vi "SPD.HV_Bias SubTest.vi"(0 "SPD.Stand Ctrl in":T3 {"spdDeviceSession"."hidSPD.Controller"."HV_bias" format="%#_6p, V"; "spdDeviceSession"."hidSPD.Controller"."TSet" format="%#_6p, DegC"}, 1 "Comparison Mode":T2, 5 "HV_values":dbl[](array[numeric]), 7 "Gate":dbl, 9 "range":T1, 11 "Error In":errorcluster, 12 "Progress":refnum<vi>, 13 "Graph":refnum<vi>) -> (4 "SPD.Stand Ctrl out":T3 {"spdDeviceSession"."hidSPD.Controller"."HV_bias" format="%#_6p, V"; "spdDeviceSession"."hidSPD.Controller"."TSet" format="%#_6p, DegC"}, 6 "last HV_bias":dbl, 8 "Clicks Count":dbl, 10 "result":bool, 15 "Error Out":errorcluster)   [LabVIEW 2018]
uses:
  typedefs/SPD.Stand Ctrl.ctl
  Instruments/SPD HID Interface/hidSPDLibForLabView/LibVIs/hidSPD Controls/hidSPD Device Session.ctl
  Instruments/SPD HID Interface/hidSPDLibForLabView/LibVIs/hidSPD Controls/hidSPD Controller.ctl
  Instruments/KC705 DevBoard/typedefs/DevB.Session.ctl
  Instruments/KeySight 53230A/typedefs/FreqC.Session.ctl
  Instruments/KeySight 8164B/KeySight 8164B LAN InstrLib/typedefs/KeySight 8164B control.ctl
  Instruments/LeCroy SDA830/typedefs/LeCroy.Session.ctl
  typedefs/SPD.Events.ctl
  <vilib>/Utility/config.llb/Config Data RefNum.ctl
  SubVIs/comparison mode.ctl
  SubVIs/Min_Max.ctl
  Instruments/SPD HID Interface/hidSPDLibForLabView/LibVIs/hidSPD Controls/hidSPD Controller Setup Report.ctl
  Instruments/SPD HID Interface/hidSPDLibForLabView/LibVIs/hidSPD Write Report/hidSPD Setup Controller.vi
  Instruments/SPD HID Interface/hidSPDLibForLabView/hidSPDLibForLabView.lvlib
  Instruments/KeySight 8164B/KeySight 8164B LAN InstrLib.lvlib
  <vilib>/Utility/config.llb/NI_LVConfig.lvlib
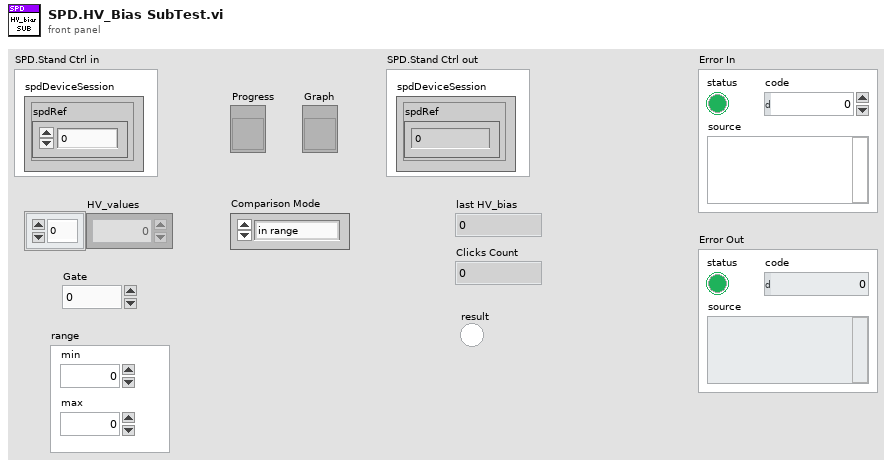
[diagram p1: front panel]
types:
  T1 = typedef "Min_Max.ctl" = cluster{"min":dbl, "max":dbl}
  T2 = typedef "comparison mode.ctl" = enum16{"in range", "bigger then min", "bigger then max", "less then min", "less then max"}
  T3 = typedef "SPD.Stand Ctrl.ctl" = cluster{"spdDeviceSession":T4, "DevBSession":T6, "FreqCSession":T7, "8164BSession":T8, "LeCroySession":T9, "Events":T10, "configFile":T11}
  T4 = typedef "hidSPDLibForLabView.lvlib/hidSPD Device Session.ctl" = cluster{"spdRef":u64, "connected":bool, "spdName":string, "hidSPD.Controller":T5}
  T5 = typedef "hidSPDLibForLabView.lvlib/hidSPD Controller.ctl" = cluster{"TSet":sgl, "HV_bias":sgl, "DDS_stb_code":u16}
  T6 = typedef "DevB.Session.ctl" = cluster{"DevBRef":refnum<visa-resource-name>, "connected":bool}
  T7 = typedef "FreqC.Session.ctl" = cluster{"FreqCRef":refnum<visa-resource-name>, "timeout":dbl, "connected":bool}
  T8 = typedef "KeySight 8164B LAN InstrLib.lvlib/KeySight 8164B control.ctl" = cluster{"Connection ID":refnum<k5>, "Connected":bool, "Info":string, "Slots Info":string[]}
  T9 = typedef "LeCroy.Session.ctl" = cluster{"LeCroySession":refnum<visa-resource-name>, "connected":bool}
  T10 = typedef "SPD.Events.ctl" = cluster{"DCRTest":refnum<user-event>, "Stop":refnum<user-event>}
  T11 = typedef "NI_LVConfig.lvlib/Config Data RefNum.ctl" = refnum<k1>
  T12 = typedef "hidSPDLibForLabView.lvlib/hidSPD Controller Setup Report.ctl" = cluster{"TSet":sgl, "HV_bias":sgl, "DDS_stb_code":u16, "SPD_reset":u16, "MCU_reset":u16}
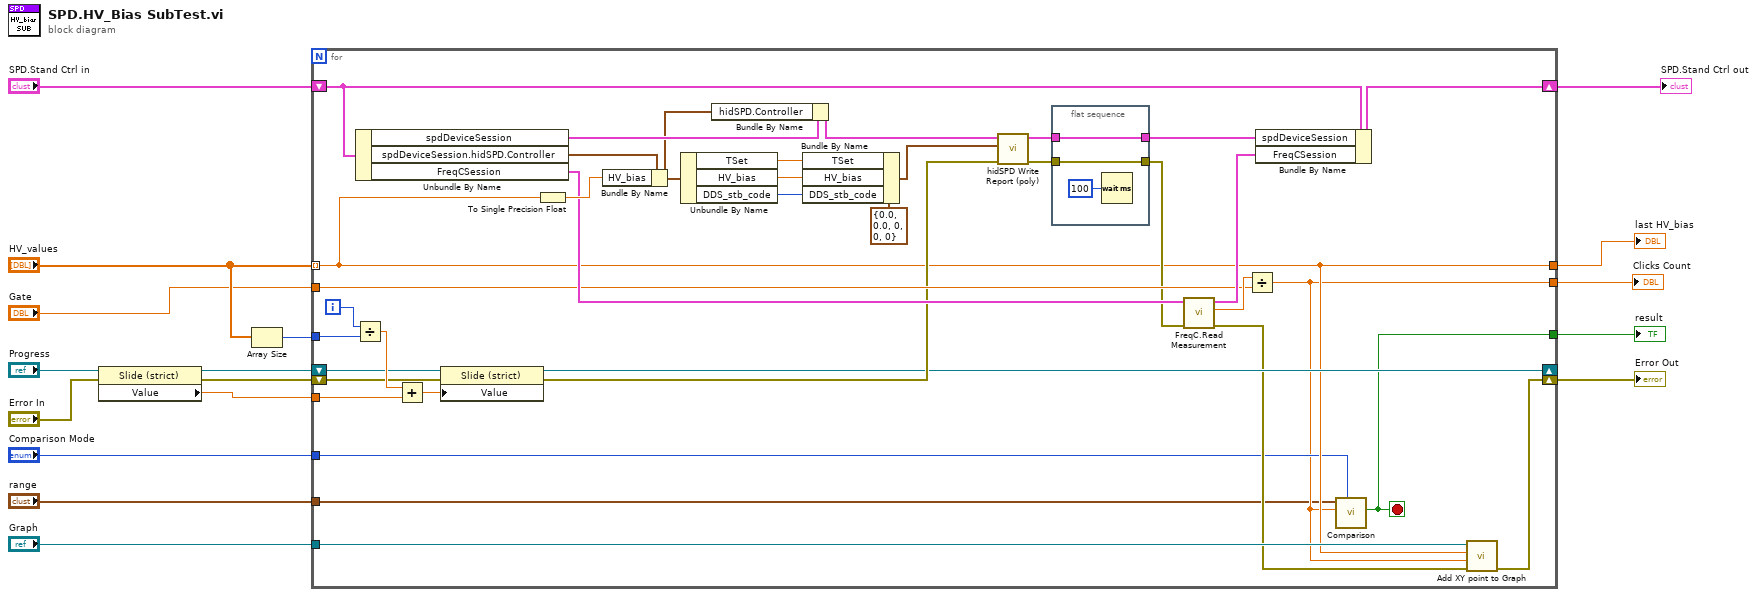
[diagram p0: block diagram]
diagram:
  n1 = property class="Slide (strict)"(reference="Progress", error in="Error In") -> (reference out=w8:refnum<vi>, error out=w6:errorcluster, "Value"=w5:dbl)
  n2 = Array Size(array="HV_values") -> (size(s)=w13:i32)
  n3 = for {
    shift-right: [w25] -> w15
    shift-left: w6 -> [w32]
    shift-right: [w43] -> w16
    shift-left: "SPD.Stand Ctrl in" -> [w47]
    tunnel: "HV_values" -> [w27] mode=indexing
    tunnel: "Gate" -> [w39]
    tunnel: [w24] -> w4
    tunnel: [w27] -> w2
    tunnel: w13 -> [w34]
    shift-right: [w30] -> _
    shift-left: w8 -> [w29]
    tunnel: "Graph" -> [w28]
    tunnel: [w22] -> w3
    tunnel: "Comparison Mode" -> [w23]
    tunnel: w5 -> [w20]
    tunnel: "range" -> [w18]
    i -> [w19]
    stop <- w24 stop-if-true
    n4 = Divide(x=w19, y=w34) -> (x/y=w33:dbl)
    n5 = Unbundle By Name(w47) -> ("spdDeviceSession"=w54:T4, "spdDeviceSession.hidSPD.Controller"=w52:T5, "FreqCSession"=w41:T7)
    n6 = Add(x=w33, y=w20) -> (x+y=w21:dbl)
    n7 = property class="Slide (strict)"(reference=w29, error in=w32, "Value"=w21) -> (reference out=w30:refnum<vi>, error out=w31:errorcluster)
    n8 = To Single Precision Float(number=w27) -> (single precision float=w42:sgl)
    n9 = Bundle By Name(cluster=w52, "HV_bias"=w42) -> (w45:T5)
    n10 = Unbundle By Name(w45) -> ("TSet"=w51:sgl, "HV_bias"=w50:sgl, "DDS_stb_code"=w49:u16)
    n11 = Bundle By Name(cluster=w54, "hidSPD.Controller"=w45) -> (w46:T4)
    n12 = Bundle By Name(cluster=T12 {"TSet"=0.0, "HV_bias"=0.0, "DDS_stb_code"=0, "SPD_reset"=0, "MCU_reset"=0} ("hidSPD Controller Setup report"), "TSet"=w51, "HV_bias"=w50, "DDS_stb_code"=w49) -> (w48:T12)
    n13 = call-poly "hidSPD Write Report (poly).vi"("error in (no error)"=w31, "hidSPD Controller Setup report"=w48, "spdDevSession in"=w46) -> ("error out"=w37:errorcluster, "spdDevSession out"=w38:T4)  [unwired: 7 in]
    n14 = flat-sequence {
      tunnel: [w57] -> w35
      tunnel: w38 -> [w57]
      tunnel: [w56] -> w36
      tunnel: w37 -> [w56]
      frame #0 {
        n15 = Wait (ms)(milliseconds to wait=u32 100) -> ()  [unwired: 1 out]
      }
    }
    n16 = call "FreqC.Read Measurement.vi"("error In"=w36, "FreqC Session in"=w41) -> ("error out"=w26:errorcluster, "Measurement"=w40:dbl, "FreqC Session out"=w44:T7)  [unwired: 7 in]
    n17 = Divide(x=w40, y=w39) -> (x/y=w22:dbl)
    n18 = Bundle By Name(cluster=w47, "spdDeviceSession"=w35, "FreqCSession"=w44) -> (w43:T3)
    n19 = call "Comparison.vi"("Comparison Mode"=w23, "value"=w22, "minMax"=w18) -> ("result"=w24:bool)  [unwired: 8 in]
    n20 = call "Add XY point to Graph.vi"("error in (no error)"=w26, "Y"=w22, "X"=w27, "Graph in"=w28) -> ("error out"=w25:errorcluster)  [unwired: 6 in, 1 out]
  }
  "SPD.Stand Ctrl out" <- w16
  "Error Out" <- w15
  "result" <- w4
  "Clicks Count" <- w3
  "last HV_bias" <- w2
